vi "MICSD Calibrate.vi"(0 "VISA Resource Name":refnum<visa-resource-name>, 1 "Execute on Remote?(F)":bool, 5 "CalSelect1":u8 format="%.0x", 7 "CalSelect2":u8 format="%.0x", 9 "Channel":i8, 11 "error in (no error)":errorcluster) -> (4 "dup VISA Resource Name":refnum<visa-resource-name>, 15 "error out":errorcluster)   [LabVIEW 2020]
uses:
  <vilib>/Instr/_visa.llb/VISA Configure Serial Port (Instr).vi
panel:
  # "* defines to select group 1 cals */\nCAL_WAKEUP_STROBE_OSC     0x01\nCAL_TX_IF_OSC             0x02\nCAL_FM_DETECT_AND_RX_IF   0x04\nCAL_RX_ADC                0x08\nCAL_400_MHZ_TX_102        0x10  \nCAL_400_MHZ_RX_102        0x20\nCAL_400_MHZ_ANT           0x40\nCAL_24_MHZ_CRYSTAL_OSC    0x80\n/* defines to select group 2 cals/\nCAL_2_MHZ_OSC_102         (0x01 << 8) \nCAL_LNA_FREQ_102          (0x02 << 8)"
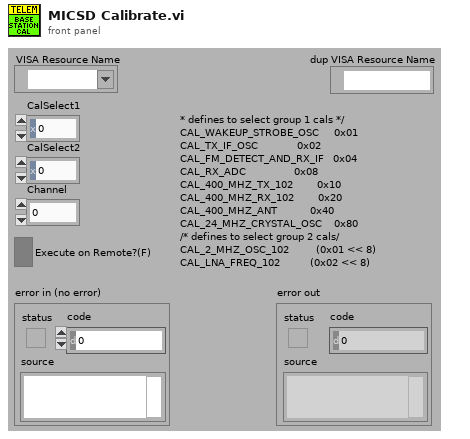
[diagram p1: front panel]
types:
  T1 = cluster{"Command Token":u8, "Length":u16, "Pack Data":u8[]}
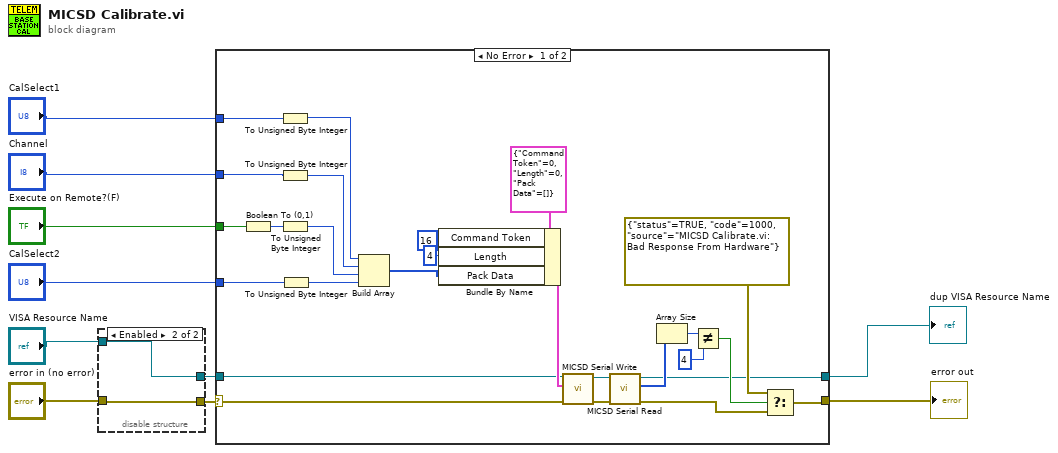
[diagram p0: block diagram]
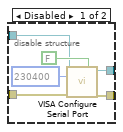
[diagram p2: hidden frame]
diagram:
  n1 = disable-structure shown="Enabled" {
    disable-tunnel: [w14 w17] -> w10
    disable-tunnel: [w13 w18] -> w9
    disable-tunnel: "VISA Resource Name" -> [w12 w18]
    disable-tunnel: "error in (no error)" -> [w11 w17]
    frame Disabled {
      n2 = call-poly "VISA Configure Serial Port"("VISA resource name"=w12, "Enable Termination\nChar (T)"=FALSE ("Enable Termination\nChar (T)"), "baud rate (9600)"=u32 230400, "error in (no error)"=w11) -> ("VISA resource name out"=w13:refnum<visa-resource-name>, "error out"=w14:errorcluster)  [unwired: 10 in]
    }
    frame Enabled {
    }
  }
  n3 = case shown="No Error" w10 {
    selector: w10 -> [w39 w45]
    tunnel: w9 -> [w40 w46]
    tunnel: "CalSelect1" -> [w30 _]
    tunnel: "Channel" -> [w29 _]
    tunnel: "Execute on Remote?(F)" -> [w38 _]
    tunnel: [w19 w45] -> w5
    tunnel: [w20 w46] -> w6
    tunnel: "CalSelect2" -> [w27 _]
    frame No Error {
      n4 = Boolean To (0,1)(Boolean=w38) -> (0, 1=w37:i16)
      n5 = To Unsigned Byte Integer(number=w30) -> (unsigned 8bit integer=w36:u8)
      n6 = To Unsigned Byte Integer(number=w29) -> (unsigned 8bit integer=w35:u8)
      n7 = To Unsigned Byte Integer(number=w37) -> (unsigned 8bit integer=w34:u8)
      n8 = To Unsigned Byte Integer(number=w27) -> (unsigned 8bit integer=w28:u8)
      n9 = Build Array(w36, w35, w34, w28) -> (w33:u8[])
      n10 = Bundle By Name(cluster=T1 {"Command Token"=0, "Length"=0, "Pack Data"=[]} ("Write Data"), "Command Token"=u8 16, "Length"=u16 4, "Pack Data"=w33) -> (w44:T1)
      n11 = call "MICSD Serial Write.vi"("error in (no error)"=w39, "Write Data"=w44, "VISA Resource Name"=w40) -> ("error out"=w31:errorcluster, "DUP Visa Resource Name"=w32:refnum<visa-resource-name>)  [unwired: 7 in]
      n12 = call "MICSD Serial Read.vi"("error in (no error)"=w31, "VISA Resource Name"=w32) -> ("error out"=w22:errorcluster, "Read Data"=w21:u8[], "DUP Visa Resource Name"=w20:refnum<visa-resource-name>)  [unwired: 7 in]
      n13 = Array Size(array=w21) -> (size(s)=w25:i32)
      n14 = Not Equal?(x=w25, y=4) -> (x != y?=w24:bool)
      n15 = Select(t=errorcluster {"status"=TRUE, "code"=1000, "source"="MICSD Calibrate.vi:  Bad Response From Hardware"} ("error IO"), s=w24, f=w22) -> (s? t:f=w19:errorcluster)
    }
    frame Error {
    }
  }
  "dup VISA Resource Name" <- w6
  "error out" <- w5
